vi "Reset Device.vi"(8 "error in (no error)":errorcluster, 10 "Reset":bool, 11 "CS++DeviceActor in":refnum<class "CS++DeviceActor.lvclass">) -> (0 "error out":errorcluster, 3 "CS++DeviceActor out":refnum<class "CS++DeviceActor.lvclass">)   [LabVIEW 2016, in "CS++DeviceActor.lvlib" / "CS++DeviceActor.lvclass"]
doc: "Perform reset of device."
uses:
  CS++DeviceActor.lvclass
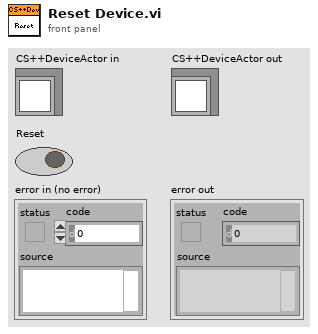
[diagram p1: front panel]
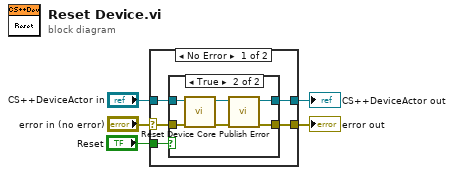
[diagram p0: block diagram]
diagram:
  n1 = case shown="No Error" "error in (no error)" {
    selector: "error in (no error)" -> [w8 w20]
    tunnel: [w7 w20] -> w4
    tunnel: [w9 w19] -> w2
    tunnel: "CS++DeviceActor in" -> [w10 w19]
    tunnel: "Reset" -> [w6 _]
    frame No Error {
      n2 = case shown="True" w6 {
        tunnel: w10 -> [w12 w18]
        tunnel: [w12 w14] -> w9
        tunnel: w8 -> [w11 w17]
        tunnel: [w11 w13] -> w7
        frame False {
        }
        frame True {
          n3 = call-dynamic "Reset Device Core.vi"("error in (no error)"=w17, "CS++DeviceActor in"=w18) -> ("error out"=w15:errorcluster, "CS++DeviceActor out"=w16:refnum<class "CS++DeviceActor.lvclass">)  [unwired: 8 in]
          n4 = call "Publish Error.vi"("error in (no error)"=w15, "CS++DeviceActor in"=w16) -> ("error out"=w13:errorcluster, "CS++DeviceActor out"=w14:refnum<class "CS++DeviceActor.lvclass">)  [unwired: 8 in]
        }
      }
    }
    frame Error {
    }
  }
  "error out" <- w4
  "CS++DeviceActor out" <- w2
